vi "Main Panel.vi"(8 "error in (no error)":errorcluster) -> (0 "error out":errorcluster)   [LabVIEW 2014]
uses:
  Type'def/UPH Config.ctl
  SubVI's/VISA/Ctr/VISA Ctr.ctl
  Type'def/MainCtr.ctl
  Type'def/Main Ctr Ref.ctl
  Type'def/User Login.ctl
  <vilib>/addons/database/Connection.llb/Conn ObjectReference.ctl
  <vilib>/addons/database/NI_Database_API.lvlib
  SubVI's/Database/Ctr/Constr.ctl
  SubVI's/Database/Ctr/Conneect State.ctl
  Type'def/DB Query.ctl
  Type'def/Main FTT.ctl
  SubVI's/Simatic S7/Function/Write/Write Sigle Data/Write Sigle Bool.vi
  SubVI's/Simatic S7/Simatic S7.lvlib
  <vilib>/addons/database/_DB Variant To Data/Database Variant To Data.xnode
  Type'def/FTT Display Type.ctl
panel:
  out "ArrayStr out":string[](array[string])
  in  "Login":bool
  out "Login":T1 caption="用户登录信息"
  out "Date&Time":string
  in  "Exit":bool
  in  "Config":bool
  in  "Query DB":bool
  in  "Main Panel":bool
  in  "Table":enum32{"Main", "Database", "Config"}(tab)
  in  "Error Table":i32(listbox)
  out "Display":T2
  in  "DB Dispaly":T3 {"StartTime" format="%<%Y/%m/%d %H:%M>T"; "EndTime" format="%<%Y/%m/%d %H:%M>T"}
  in  "FTT_Submit":bool
  out "IP Address":string[](array[string])
  in  "Scaner":bool
  in  "Shield Signe":bool
  in  "UPH":bool
  in  "Modfy TV":bool
  # "Inalfa roof systems(Shanghai) CO.LT"
  # "Plan/Targe(%)"
  # "Taget/Actual"
  # "FTT/FTT(%)"
  # "Repaired/Reject"
  # "/"
  # "/"
  # "/"
  # "/"
  # "硬件配置"
  # "参数配置"
  # "其他配置"
  # "当前系统CPU地址"
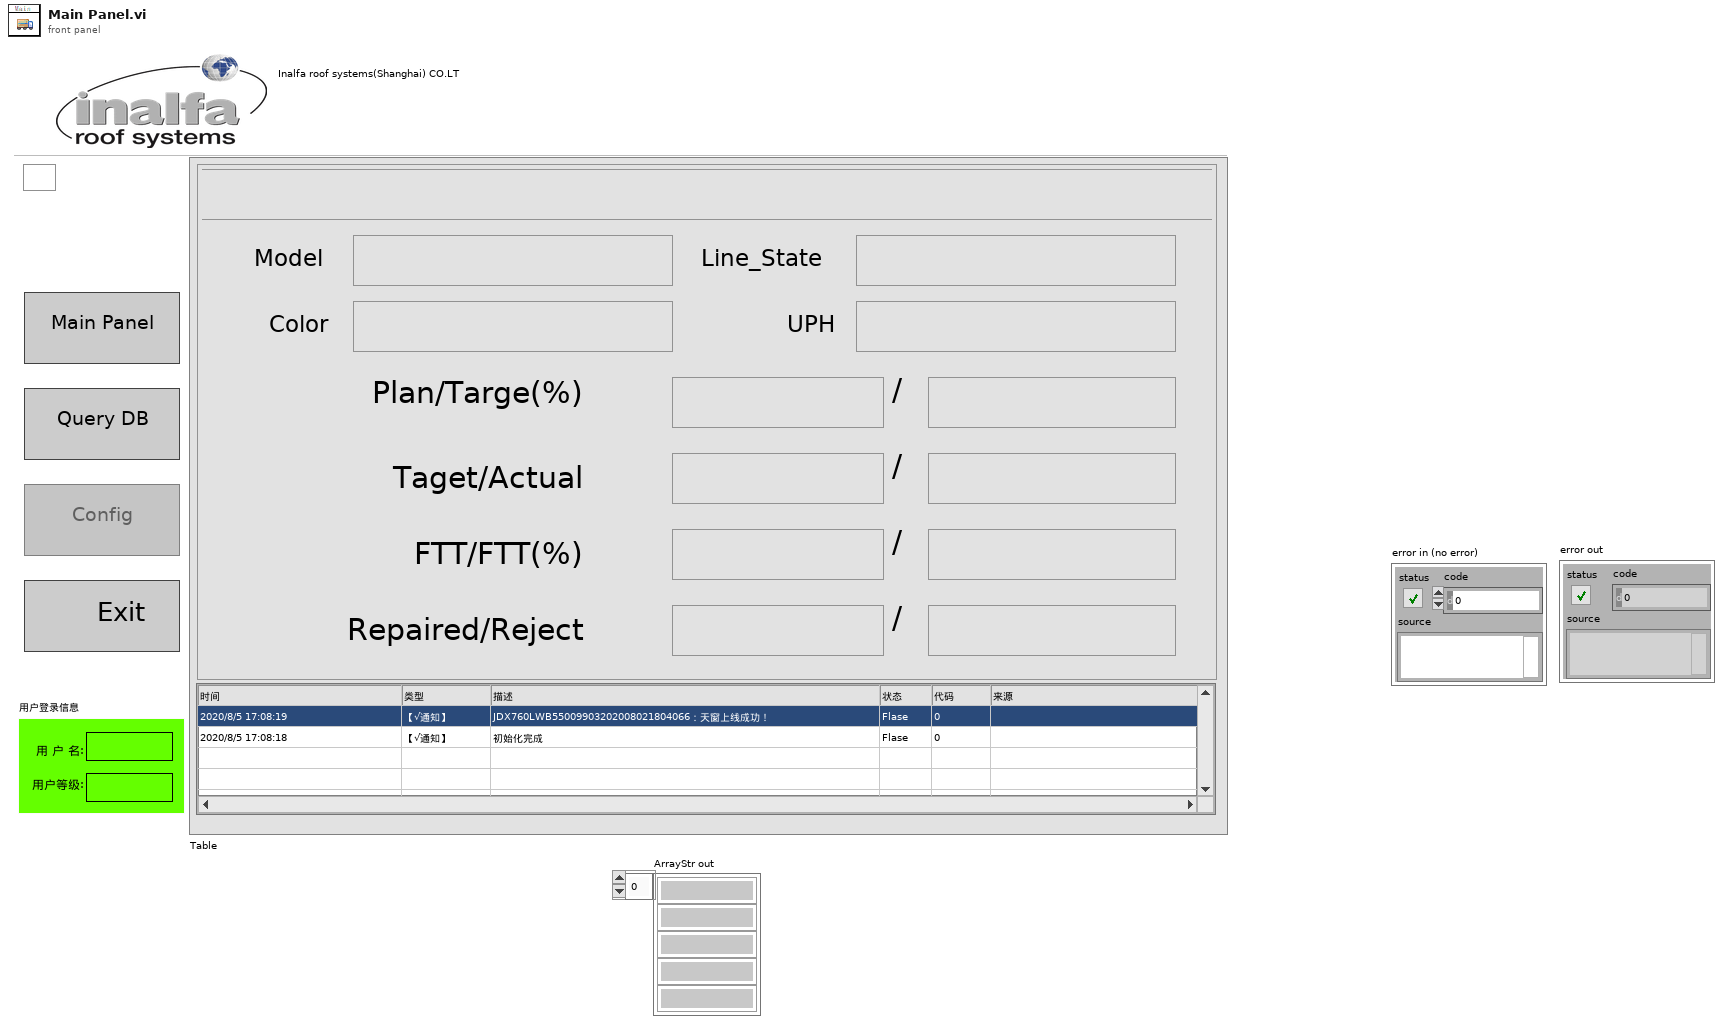
[diagram p1: front panel]
types:
  T1 = typedef "User Login.ctl" = cluster{"User":string, "Grade":string}
  T2 = typedef "Main FTT.ctl" = cluster{"Line_Name":string, "Model":string, "Line_State":string, "Color":string, "UPH":string, "Plan":string, "Target Rate":string, "Target":string, "Actual":string, "FTT":string, "FTT Rate":string, "Repaired":string, "Reject":string}
  T3 = cluster{"Export":bool, "Query":bool, "Station.No":string, "EndTime":timestamp, "StartTime":timestamp, "FTT":cluster{"FTT":string, "OutLine":string, "FTT Rata":string}, "TableName":string, "List":string[][], "Station":bool, "QTime":enum32{"Online", "Outline"}}
  T4 = typedef "MainCtr.ctl" = cluster{"Tite":string, "Base path":path, "Table":cluster{"Table":string, "alias":string}[], "Stations":cluster{"Stations":string, "alias":string}[], "Shield Array":bool[], "UPHs":T5[], "VISA":T6, "Path":cluster{"roof":path, "Config":path, "Png":path}, "Ctr":T7, "Login":T1, "information":cluster{"cause":string, "Type":enum16{"Inform", "Warning", "Alarm"}, "code":i32, "Suroce":string, "Status":bool}, "Local DB":cluster{"Connstr":string, "Database":T8}, "Remote DB":cluster{"Connstr":string, "Database":T8}, "FTT TV":string, "ExchangeTime":i32, "NVH":string, "EOL Path":path}
  T5 = typedef "UPH Config.ctl" = cluster{"Line_No":string, "Model":string, "B_UPH ":i16, "S_UPH  ":i16, "Class":enum16{"Big", "Small"}}
  T6 = typedef "VISA Ctr.ctl" = cluster{"VISA":refnum<visa-resource-name>, "baud rate":u32, "data bits":u16, "parity":enum16{"None", "Odd", "Even", "Mark", "Space"}, "stop bits":u16, "flow control":u16}
  T7 = typedef "Main Ctr Ref.ctl" = cluster{"DB Dispaly":refnum<vi>, "Error Table":refnum<vi>, "Display":refnum<vi>, "Login":refnum<vi>, "Exit":refnum<vi>, "FTT_Submit":refnum<vi>}
  T8 = typedef "Conneect State.ctl" = cluster{"Constr":T9, "conn ref":T10, "State":bool}
  T9 = typedef "Constr.ctl" = cluster{"Driver":string, "Server":string, "User":string, "Pwd":string, "Database":string}
  T10 = typedef "NI_Database_API.lvlib/Conn ObjectReference.ctl" = refnum<k1>
  T11 = enum8{"Enabled", "Disabled", "Disabled and Grayed Out"}
  T12 = typedef "DB Query.ctl" = cluster{"Export":bool, "Query":bool, "Station.No":string, "EndTime":timestamp, "StartTime":timestamp, "FTT":cluster{"FTT":string, "OutLine":string, "FTT Rata":string}, "TableName":string, "List":string[][], "Station":bool, "QTime":enum32{"Online", "Outline"}}
  T13 = typedef "FTT Display Type.ctl" = cluster{"Line.No":string, "Model":string, "Color":string, "UPH":dbl, "Plan":dbl, "Target Rate":dbl, "Target ":dbl, "Actual":dbl, "FTT":dbl, "FTT Rate":dbl, "Repaired":dbl, "Reject":dbl, "Ouline":dbl, "Line State":string}
  T14 = cluster{"Display":T13, "Class":enum16{"Big", "Small"}}
  T15 = cluster{"cause":string, "Type":enum16{"Inform", "Warning", "Alarm"}, "code":i32, "Suroce":string, "Status":bool}
  T16 = typedef "Simatic S7.lvlib/Operation Siemens Ref.ctl" = enum16{"Init", "Add Ref", "Get Ref", "Set Error", "Close Close"}
  T17 = cluster{"Base path":path, "Config path":path, "Log DB Error":path}
  T18 = cluster{"DB Dispaly":refnum<vi>, "Error Table":refnum<vi>, "Display":refnum<vi>, "Login":refnum<vi>, "Exit":refnum<vi>, "FTT_Submit":refnum<vi>}
  T19 = cluster{"Username":string, "GradeStr":string, "Grade":u32}
  T20 = typedef "Simatic S7.lvlib/Siemens Ref.ctl" = cluster{"IP Address ":string, "Conn ID":refnum<k5>, "Timeout ms":i32, "Status":bool, "Slot":u16, "Rack":u16}
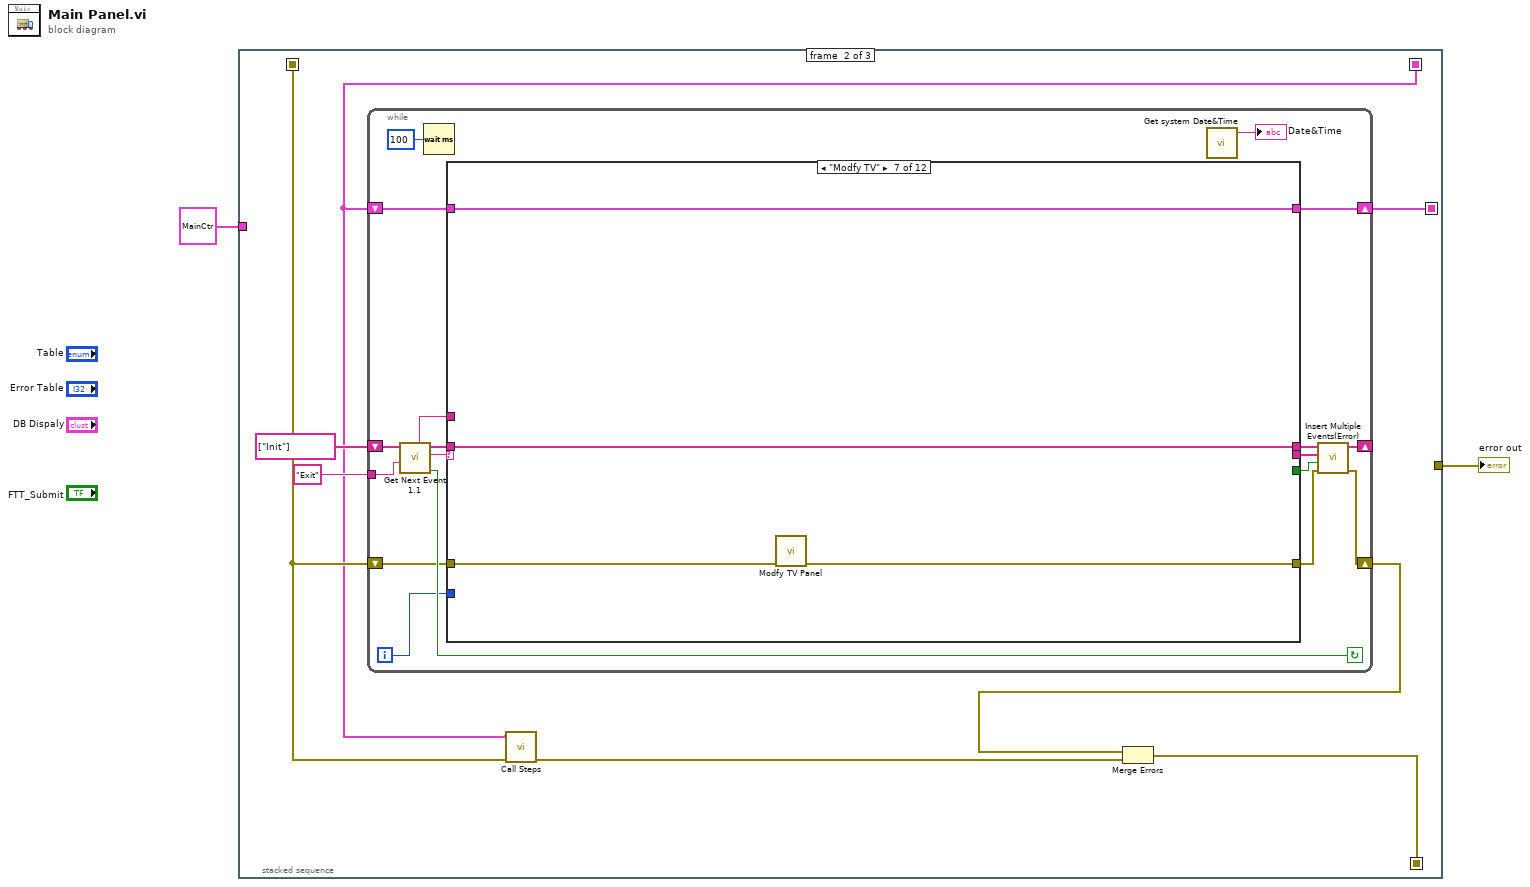
[diagram p0: block diagram]
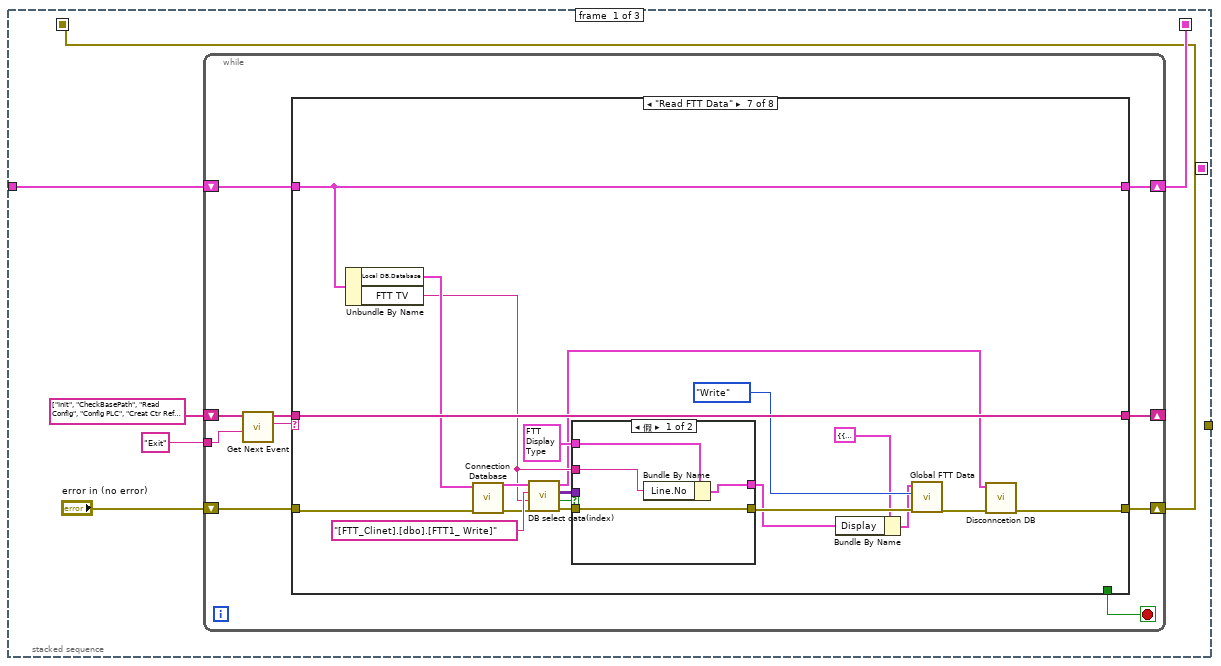
[diagram p2: hidden frame]
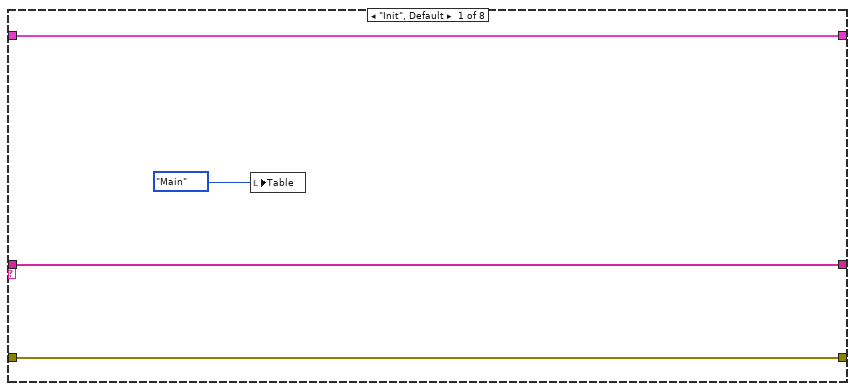
[diagram p3: hidden frame]
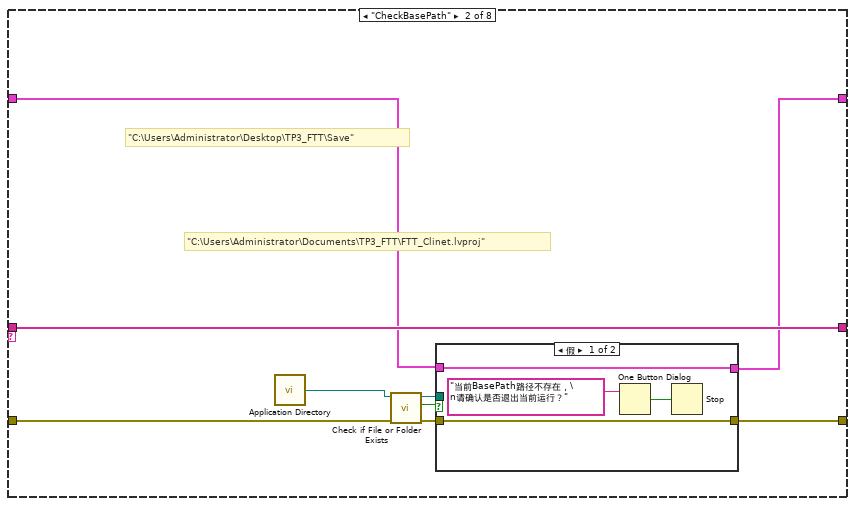
[diagram p4: hidden frame]
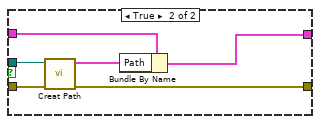
[diagram p5: hidden frame]
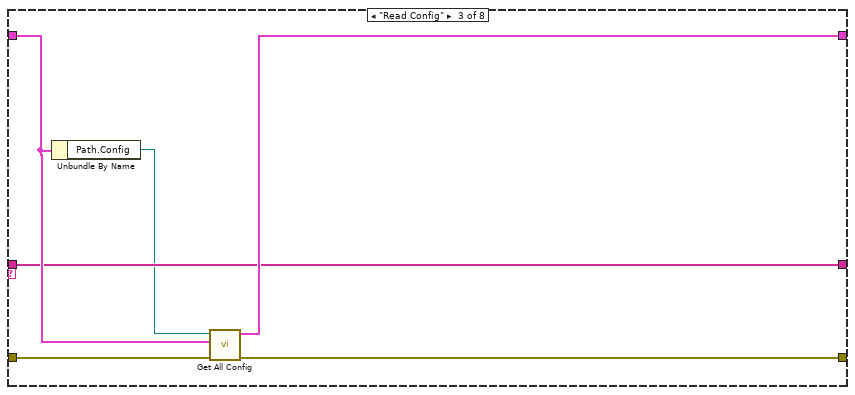
[diagram p6: hidden frame]
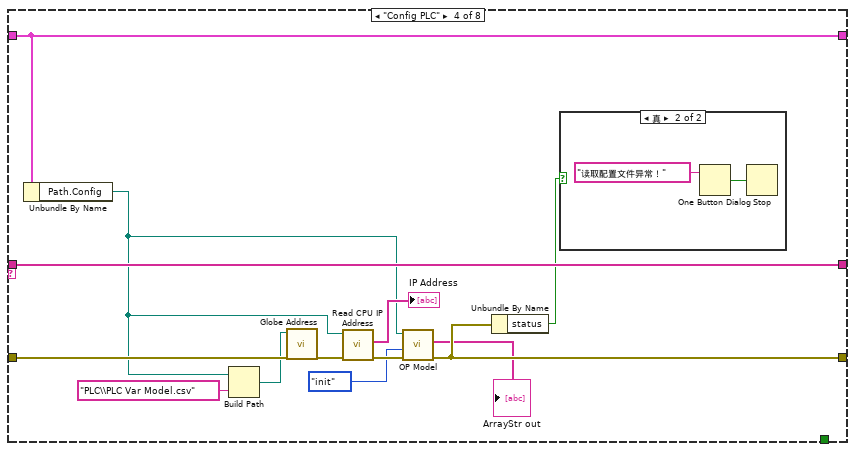
[diagram p7: hidden frame]
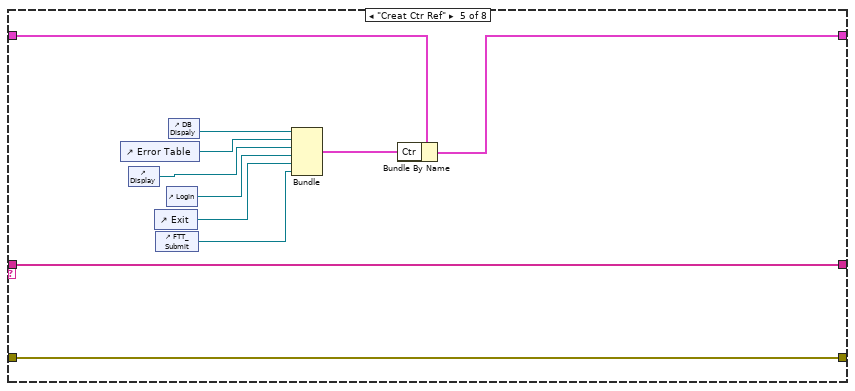
[diagram p9: hidden frame]
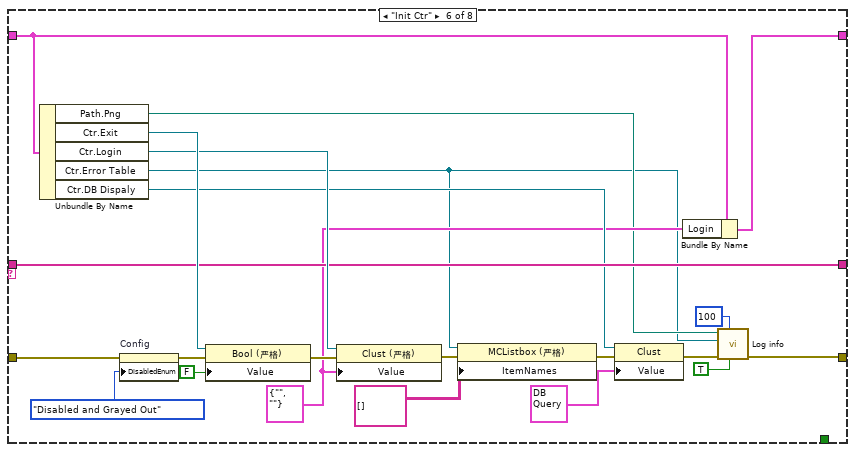
[diagram p10: hidden frame]
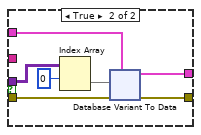
[diagram p11: hidden frame]
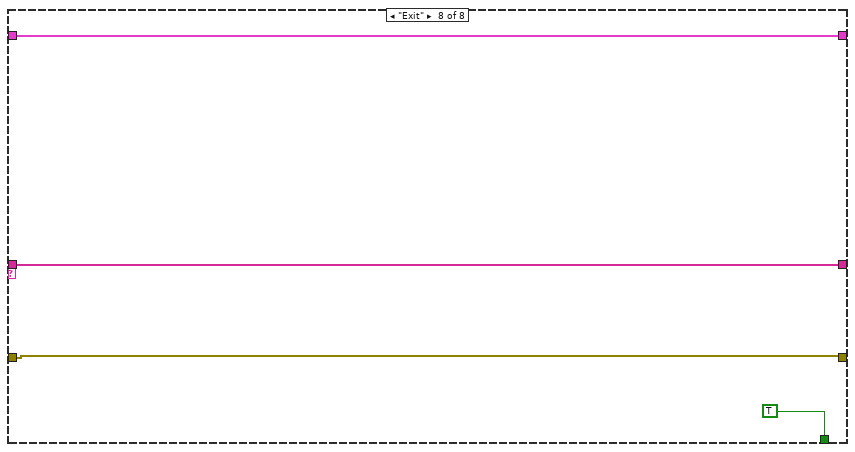
[diagram p12: hidden frame]
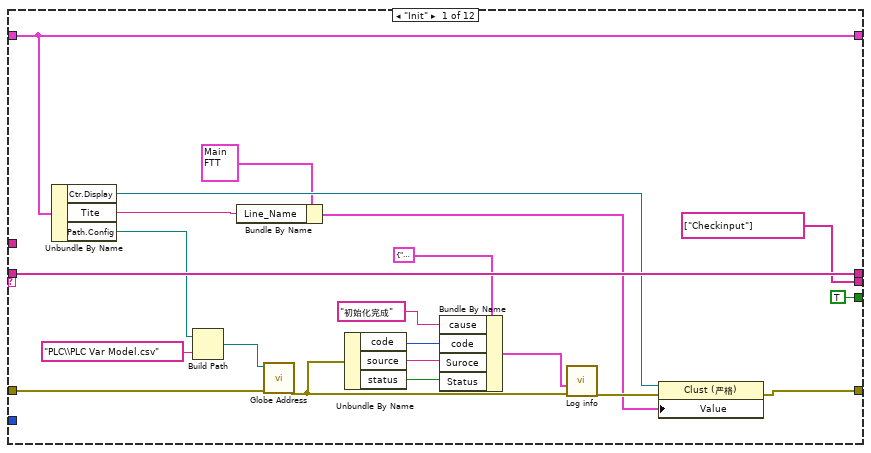
[diagram p13: hidden frame]
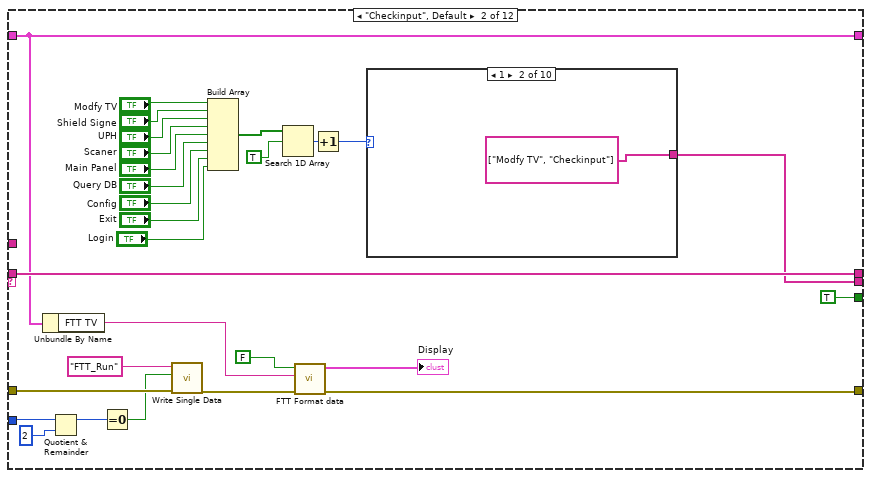
[diagram p14: hidden frame]
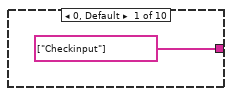
[diagram p15: hidden frame]
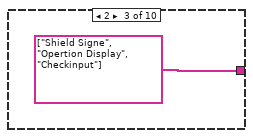
[diagram p16: hidden frame]
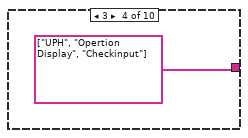
[diagram p17: hidden frame]
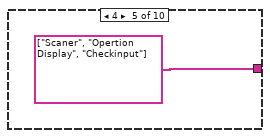
[diagram p18: hidden frame]
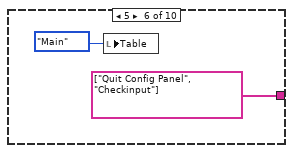
[diagram p19: hidden frame]
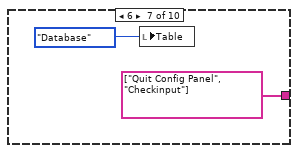
[diagram p20: hidden frame]
diagram:
  n1 = stacked-sequence {
    seq-local: [w4 _ _] -> [_ w569 _]
    seq-local: [w3 _ _] -> [_ w574 _]
    seq-local: [_ w571 _] -> [_ _ w768]
    seq-local: [_ w570 _] -> [_ _ _]
    tunnel: T4 {"Tite"="", "Base path"=path "", "Table"=[], "Stations"=[], "Shield Array"=[], "UPHs"=[], "VISA"={"VISA"="", "baud rate"=9600, "data bits"=8, "parity"=enum."None", "stop bits"=10, "flow control"=0}, "Path"={"roof"=path "", "Config"=path "", "Png"=path ""}, "Ctr"={"DB Dispaly"=refnum, "Error Table"=refnum, "Display"=refnum, "Login"=refnum, "Exit"=refnum, "FTT_Submit"=refnum}, "Login"={"User"="", "Grade"=""}, "information"={"cause"="", "Type"=enum."Inform", "code"=0, "Suroce"="", "Status"=FALSE}, "Local DB"={"Connstr"="", "Database"={"Constr"={"Driver"="", "Server"="", "User"="", "Pwd"="", "Database"=""}, "conn ref"=refnum, "State"=FALSE}}, "Remote DB"={"Connstr"="", "Database"={"Constr"={"Driver"="", "Server"="", "User"="", "Pwd"="", "Database"=""}, "conn ref"=refnum, "State"=FALSE}}, "FTT TV"="", "ExchangeTime"=0, "NVH"="", "EOL Path"=path ""} ("Cluster") -> [w6 _ _]
    tunnel: [_ _ w762] -> w1
    frame #0 {
      n2 = while {
        shift-right: [w13] -> _
        shift-left: string[] ["Init", "CheckBasePath", "Read Config", "Config PLC", "Creat Ctr Ref", "Read FTT Data", "Init Ctr", "Exit"] -> [w18]
        tunnel: "Exit" ("Exit Event") -> [w15]
        shift-right: [w10] -> w4
        shift-left: w6 -> [w14]
        shift-right: [w11] -> w3
        shift-left: "error in (no error)" -> [w12]
        stop <- w9 stop-if-true
        n3 = call "Get Next Event.vi"("Exit Event"=w15, "event queue in"=w18) -> ("next event"=w17:string, "event queue out"=w16:string[])  [unwired: 3 in, 1 out]
        n4 = case shown="\"Read FTT Data\"" w17 {
          tunnel: w16 -> [w21 w31 w44 w55 w73 w89 w115 w567]
          tunnel: w14 -> [w22 w26 w46 w59 w67 w85 w99 w566]
          tunnel: [w21 w31 w44 w55 w73 w89 w115 w567] -> w13
          tunnel: w12 -> [w20 w30 w47 w58 w72 w76 w106 w565]
          tunnel: [w20 w25 w42 w51 w72 w81 w100 w565] -> w11
          tunnel: [w22 w24 w45 w59 w66 w84 w99 w566] -> w10
          tunnel: [_ _ _ _ _ _ _ TRUE] -> w9
          frame "Init", Default {
            n5 = local write "Table"(enum32{"Main", "Database", "Config"}."Main" ("Table")) -> ()
          }
          frame "CheckBasePath" {
            # "\"C:\\Users\\Administrator\\Documents\\TP3_FTT\\FTT_Clinet.lvproj\""
            # "\"C:\\Users\\Administrator\\Desktop\\TP3_FTT\\Save\""
            n6 = call <vilib>:"Application Directory.vi"() -> ("Application Directory"=w23:path)
            n7 = call <vilib>:"Check if File or Folder Exists.vi"("error in (no error)"=w30, "path"=w23) -> ("error out"=w28:errorcluster, "file or folder exists?"=w29:bool, "dup path"=w27:path)  [unwired: 7 in]
            n8 = case shown="假" w29 {
              tunnel: w28 -> [w35 w41]
              tunnel: w27 -> [_ w40]
              tunnel: w26 -> [w34 w39]
              tunnel: [w35 w37] -> w25
              tunnel: [w34 w36] -> w24
              frame False {
                n9 = One Button Dialog(message="当前BasePath路径不存在，\n请确认是否退出当前运行？") -> (true=w33:bool)  [unwired: 1 in]
                n10 = Stop(stop? (T)=w33) -> ()
              }
              frame True {
                n11 = call "Creat Path.vi"("error in (no error)"=w41, "base path"=w40) -> ("error out"=w37:errorcluster, "output cluster"=w38:T17)  [unwired: 8 in]
                n12 = Bundle By Name(cluster=w39, "Path"=w38) -> (w36:T4)
              }
            }
          }
          frame "Read Config" {
            n13 = Unbundle By Name(w46) -> ("Path.Config"=w43:path)
            n14 = call "Get All Config.vi"("error in (no error)"=w47, "Main Ctr in"=w46, "Base Path"=w43) -> ("error out"=w42:errorcluster, "Cluster"=w45:T4)  [unwired: 7 in]
          }
          frame "Config PLC" {
            n15 = Unbundle By Name(w59) -> ("Path.Config"=w49:path)
            n16 = Build Path(base path=w49, name or relative path="PLC\\PLC Var Model.csv") -> (appended path=w57:path)
            n17 = call "Globe Address.vi"("error in (no error)"=w58, "file path (dialog if empty)"=w57) -> ("error out"=w56:errorcluster)  [unwired: 6 in, 3 out]
            n18 = call "Read CPU IP Address.vi"("error in (no error)"=w56, "base path"=w49) -> ("error out"=w52:errorcluster, "IP Address"=→"IP Address":string[])  [unwired: 7 in, 1 out]
            n19 = call "OP Model.vi"("error in (no error)"=w52, "Enum"=enum16{"init", "Read", "Write"}."init", "Path"=w49) -> ("error out"=w51:errorcluster, "ArrayStr out"=→"ArrayStr out":string[])  [unwired: 6 in, 1 out]
            n20 = Unbundle By Name(w51) -> ("status"=w53:bool)
            n21 = case shown="真" w53 {
              frame False {
              }
              frame True {
                n22 = One Button Dialog(message="读取配置文件异常！") -> (true=w61:bool)  [unwired: 1 in]
                n23 = Stop(stop? (T)=w61) -> ()
              }
            }
          }
          frame "Creat Ctr Ref" {
            n24 = control-ref of="Error Table"() -> (w69:refnum<vi>)
            n25 = control-ref of="Display"() -> (w65:refnum<vi>)
            n26 = control-ref of="Exit"() -> (w71:refnum<vi>)
            n27 = control-ref of="FTT_Submit"() -> (w64:refnum<vi>)
            n28 = control-ref of="Login"() -> (w70:refnum<vi>)
            n29 = control-ref of="DB Dispaly"() -> (w68:refnum<vi>)
            n30 = Bundle("DB Dispaly"=w68, "Error Table"=w69, "Display"=w65, "Login"=w70, "Exit"=w71, "FTT_Submit"=w64) -> (w63:T18)  [unwired: 1 in]
            n31 = Bundle By Name(cluster=w67, "Ctr"=w63) -> (w66:T4)
          }
          frame "Init Ctr" {
            w83 = T1 {"User"="", "Grade"=""} ("Value")
            n32 = Unbundle By Name(w85) -> ("Path.Png"=w80:path, "Ctr.Exit"=w95:refnum<vi>, "Ctr.Login"=w92:refnum<vi>, "Ctr.Error Table"=w79:refnum<vi>, "Ctr.DB Dispaly"=w87:refnum<vi>)
            n33 = property on="Config" class="Bool"(error in=w76, "DisabledEnum"=T11."Disabled and Grayed Out" ("Disabled")) -> (error out=w75:errorcluster)  [unwired: 1 in, 1 out]
            n34 = property class="Bool (严格)"(reference=w95, error in=w75, "Value"=FALSE) -> (error out=w93:errorcluster)  [unwired: 1 out]
            n35 = property class="Clust (严格)"(reference=w92, error in=w93, "Value"=w83) -> (error out=w91:errorcluster)  [unwired: 1 out]
            n36 = property class="MCListbox (严格)"(reference=w79, error in=w91, "ItemNames"=string[][] [] ("Value")) -> (error out=w88:errorcluster)  [unwired: 1 out]
            n37 = property class="Clust"(reference=w87, error in=w88, "Value"=T12 {"Export"=FALSE, "Query"=FALSE, "Station.No"="", "EndTime"=timestamp(0 s since 1904-01-01), "StartTime"=timestamp(0 s since 1904-01-01), "FTT"={"FTT"="", "OutLine"="", "FTT Rata"=""}, "TableName"="", "List"=[], "Station"=FALSE, "QTime"=enum."Online"} ("DB Dispaly")) -> (error out=w82:errorcluster)  [unwired: 1 out]
            n38 = Bundle By Name(cluster=w85, "Login"=w83) -> (w84:T4)
            n39 = call "Log info.vi"("Ref ?"=TRUE, "Rows"=100, "error in (no error)"=w82, "MCListbox引用句柄"=w79, "Base"=w80) -> ("error out"=w81:errorcluster)  [unwired: 5 in, 1 out]
          }
          frame "Read FTT Data" {
            n40 = Unbundle By Name(w99) -> ("Local DB.Database"=w107:T8, "FTT TV"=w105:string)
            n41 = call "Connection Database.vi"("error in (no error)"=w106, "Connncet State"=w107) -> ("error out"=w109:errorcluster, "Connncet State out"=w108:T8)  [unwired: 8 in]
            n42 = call "DB select data(index).vi"("error in (no error)"=w109, "Code"=w105, "Tabe"="[FTT_Clinet].[dbo].[FTT1_ Write]", "Connncet State"=w108) -> ("error out"=w112:errorcluster, "state"=w113:bool, "data"=w111:variant[][], "Connncet State out"=w101:T8)  [unwired: 4 in]
            n43 = case shown="假" w113 {
              tunnel: w112 -> [w119 w124]
              tunnel: w111 -> [_ w126]
              tunnel: T13 {"Line.No"="", "Model"="", "Color"="", "UPH"=0.0, "Plan"=0.0, "Target Rate"=0.0, "Target "=0.0, "Actual"=0.0, "FTT"=0.0, "FTT Rate"=0.0, "Repaired"=0.0, "Reject"=0.0, "Ouline"=0.0, "Line State"=""} ("Display") -> [w118 w122]
              tunnel: [w119 w121] -> w104
              tunnel: [w116 w120] -> w97
              tunnel: w105 -> [w117 _]
              frame False {
                n44 = Bundle By Name(cluster=w118, "Line.No"=w117) -> (w116:T13)
              }
              frame True {
                n45 = Index Array(array=w126, index (row)=0) -> (element=w123:variant[])  [unwired: 1 in]
                n46 = xnode "Database Variant To Data"("database variant"=w123, "error in (no error)"=w124, "type"=w122) -> ("data"=w120:T13, "error out"=w121:errorcluster)
              }
            }
            n47 = Bundle By Name(cluster=T14 {"Display"={"Line.No"="", "Model"="", "Color"="", "UPH"=0.0, "Plan"=0.0, "Target Rate"=0.0, "Target "=0.0, "Actual"=0.0, "FTT"=0.0, "FTT Rate"=0.0, "Repaired"=0.0, "Reject"=0.0, "Ouline"=0.0, "Line State"=""}, "Class"=enum."Big"} ("Display"), "Display"=w97) -> (w96:T14)
            n48 = call "Global FTT Data.vi"("error in (no error)"=w104, "Mode"=enum16{"Read", "Write"}."Write", "Display"=w96) -> ("error out"=w102:errorcluster)  [unwired: 7 in, 1 out]
            n49 = call "Disconncetion DB.vi"("error in (no error)"=w102, "Connncet State"=w101) -> ("error out"=w100:errorcluster)  [unwired: 8 in, 1 out]
          }
          frame "Exit" {
          }
        }
      }
    }
    frame #1 {
      n50 = while {
        shift-right: [w587] -> _
        shift-left: string[] ["Init"] ("event queue out") -> [w591]
        tunnel: "Exit" ("Exit Event") -> [w588]
        shift-right: [w579] -> w572
        shift-left: w574 -> [w578]
        shift-right: [w582] -> w570
        shift-left: w569 -> [w583]
        i -> [w581]
        stop <- w589 continue-if-true
        n51 = call "Get Next Event 1.1.vi"("Exit Event"=w588, "event queue in"=w591) -> ("Condition (Exit:F)"=w589:bool, "next event"=w592:string, "event queue out"=w590:string[], "Previous Event"=w577:string)  [unwired: 6 in]
        n52 = Wait (ms)(milliseconds to wait=u32 100) -> ()  [unwired: 1 out]
        n53 = case shown="\"Modfy TV\"" w592 {
          tunnel: w590 -> [w615 w643 w668 w686 w701 w711 w722 w727 w737 w746 _ _]
          tunnel: [w615 w643 w668 w686 w701 w711 w722 w727 w737 w746 _ w760] -> w586
          tunnel: [TRUE TRUE _ _ _ _ _ _ _ _ FALSE FALSE] -> w585
          tunnel: [string[] ["Checkinput"] ("event queue out") w629 _ _ _ _ _ _ _ _ string[] ["Checkinput"] ("event queue out") _] -> w584
          tunnel: w578 -> [w612 w628 w670 w685 w702 w713 w724 w726 w735 w741 w750 w757]
          tunnel: [w596 w617 w662 w678 w696 w707 w723 w726 w730 w745 w749 w753] -> w580
          tunnel: w583 -> [w595 w620 w656 w680 w692 w710 w725 w728 w736 w744 w751 w756]
          tunnel: [w595 w620 w656 w679 w691 w709 w725 w728 w736 w744 w751 w756] -> w582
          tunnel: w581 -> [_ w627 _ _ _ _ _ _ _ _ _ _]
          tunnel: w577 -> [_ _ _ _ _ _ _ _ _ _ _ _]
          frame "Init" {
            n54 = Unbundle By Name(w595) -> ("Ctr.Display"=w600:refnum<vi>, "Tite"=w598:string, "Path.Config"=w611:path)
            n55 = Build Path(base path=w611, name or relative path="PLC\\PLC Var Model.csv") -> (appended path=w610:path)
            n56 = Bundle By Name(cluster=T2 {"Line_Name"="", "Model"="", "Line_State"="", "Color"="", "UPH"="", "Plan"="", "Target Rate"="", "Target"="", "Actual"="", "FTT"="", "FTT Rate"="", "Repaired"="", "Reject"=""} ("Value"), "Line_Name"=w598) -> (w597:T2)
            n57 = call "Globe Address.vi"("error in (no error)"=w612, "file path (dialog if empty)"=w610) -> ("error out"=w606:errorcluster)  [unwired: 6 in, 3 out]
            n58 = Unbundle By Name(w606) -> ("code"=w603:i32, "source"=w604:string, "status"=w605:bool)
            n59 = Bundle By Name(cluster=T15 {"cause"="我问问", "Type"=enum."Inform", "code"=0, "Suroce"="", "Status"=FALSE} ("information"), "cause"="初始化完成" ("Suroce"), "code"=w603, "Suroce"=w604, "Status"=w605) -> (w607:T15)
            n60 = call "Log info.vi"("error in (no error)"=w606, "information"=w607) -> ("error out"=w601:errorcluster)  [unwired: 8 in, 1 out]
            n61 = property class="Clust (严格)"(reference=w600, error in=w601, "Value"=w597) -> (error out=w596:errorcluster)  [unwired: 1 out]
          }
          frame "Checkinput", Default {
            n62 = Unbundle By Name(w620) -> ("FTT TV"=w619:string)
            n63 = Quotient & Remainder(x=w627, y=2) -> (x-y*floor(x/y)=w625:i32)  [unwired: 1 out]
            n64 = Equal To 0?(x=w625) -> (x = 0?=w624:bool)
            n65 = call-poly "Write Single Data.vi"("error in (no error)"=w628, "Data"=w624, "Tags"="FTT_Run") -> ("error out"=w622:errorcluster)  [unwired: 6 in, 2 out]
            n66 = Build Array("Modfy TV", "Shield Signe", "UPH", "Scaner", "Main Panel", "Query DB", "Config", "Exit", "Login") -> (w633:bool[])
            n67 = Search 1D Array(1D array=w633, element=TRUE) -> (index of element=w631:i32)  [unwired: 1 in]
            n68 = call "FTT Format data.vi"("error in (no error)"=w622, "FTT_TV"=w619, "W/R"=FALSE) -> ("error out"=w617:errorcluster, "Display"=→"Display":T2)  [unwired: 6 in, 1 out]
            n69 = Increment(x=w631) -> (x+1=w630:i32)
            n70 = case shown="1" w630 {
              tunnel: [string[] ["Checkinput"] ("event queue out") string[] ["Modfy TV", "Checkinput"] string[] ["Shield Signe", "Opertion Display", "Checkinput"] string[] ["UPH", "Opertion Display", "Checkinput"] string[] ["Scaner", "Opertion Display", "Checkinput"] string[] ["Quit Config Panel", "Checkinput"] string[] ["Quit Config Panel", "Checkinput"] string[] ["Config Panel", "Checkinput"] string[] ["Quit"] ("event queue out") string[] ["User Log", "Checkinput"]] -> w629
              frame 0, Default {
              }
              frame 1 {
              }
              frame 2 {
              }
              frame 3 {
              }
              frame 4 {
              }
              frame 5 {
                n71 = local write "Table"(enum32{"Main", "Database", "Config"}."Main" ("Table")) -> ()
              }
              frame 6 {
                n72 = local write "Table"(enum32{"Main", "Database", "Config"}."Database" ("Table")) -> ()
              }
              frame 7 {
              }
              frame 8 {
              }
              frame 9 {
              }
            }
          }
          frame "User Log" {
            n73 = Unbundle By Name(w656) -> ("Path.Config"=w669:path)  [unwired: 1 out]
            n74 = call "User and Password.vi"("error in (no error)"=w670, "Path"=w669) -> ("error out"=w663:errorcluster, "output cluster"=w667:T19)  [unwired: 8 in]
            n75 = Unbundle By Name(w667) -> ("Username"=w666:string, "GradeStr"=w665:string, "Grade"=w661:u32)
            n76 = Greater Than 0?(x=w661) -> (x > 0?=w659:bool)
            n77 = Bundle("Username"=w666, "GradeStr"=w665) -> (→"Login":cluster{"Username":string, "GradeStr":string})  [unwired: 1 in]
            n78 = Select(t=T11."Enabled" ("Disabled"), s=w659, f=T11."Disabled and Grayed Out" ("Disabled")) -> (s? t:f=w660:T11)
            n79 = property on="Config" class="Bool"(error in=w663, "DisabledEnum"=w660) -> (error out=w662:errorcluster)  [unwired: 1 in, 1 out]
          }
          frame "UPH" {
            n80 = Unbundle By Name(w680) -> ("UPHs"=w676:T5[], "Path.Config"=w681:path)
            n81 = call "OP UPH Config.vi"("error in (no error)"=w685, "Enum"=enum16{"init", "Read", "Write"}."Read") -> ("error out"=w683:errorcluster, "UPH out"=w682:T5[])  [unwired: 7 in, 1 out]
            n82 = call "UPH Panel.vi"("error in (no error)"=w683, "Base path"=w681, "UPH in"=w682) -> ("error out"=w678:errorcluster, "UPH out"=w677:T5[])  [unwired: 7 in]
            n83 = Unbundle By Name(w678) -> ("status"=w674:bool)
            n84 = Select(t=w676, s=w674, f=w677) -> (s? t:f=w675:T5[])
            n85 = Select(t="UPH修改保存异常！", s=w674, f="UPH修改保存成功！") -> (s? t:f=w673:string)
            n86 = Bundle By Name(cluster=w680, "UPHs"=w675, "information.cause"=w673) -> (w679:T4)
          }
          frame "Scaner" {
            n87 = Unbundle By Name(w692) -> ("VISA"=w694:T6, "Path.Config"=w697:path)
            n88 = call "OP Scaner Config.vi"("error in (no error)"=w702, "Enum"=enum16{"init", "Read", "Write"}."Read") -> ("error out"=w699:errorcluster, "VISA"=w698:T6)  [unwired: 7 in, 1 out]
            n89 = call "Scaner Panel.vi"("error in (no error)"=w699, "VISA in"=w698, "Base path"=w697) -> ("error out"=w696:errorcluster, "VISA out"=w695:T6)  [unwired: 7 in]
            n90 = Unbundle By Name(w696) -> ("status"=w690:bool)
            n91 = Select(t=w694, s=w690, f=w695) -> (s? t:f=w693:T6)
            n92 = Select(t="Scaner修改保存异常！", s=w690, f="Scaner修改保存成功！") -> (s? t:f=w689:string)
            n93 = Bundle By Name(cluster=w692, "VISA"=w693, "information.cause"=w689) -> (w691:T4)
          }
          frame "Shield Signe" {
            w706 = enum16{"init", "Read", "Write"}."Read" ("Enum")
            n94 = Unbundle By Name(w710) -> ("Shield Array"=w719:bool[], "Path.Config"=w720:path, "Stations"=w704:cluster{"Stations":string, "alias":string}[])
            n95 = call "OP Shield Config.vi"("error in (no error)"=w713, "Enum"=w706) -> ("error out"=w721:errorcluster, "Shield out"=w712:u32)  [unwired: 6 in, 2 out]
            n96 = call "Ger All Station Alias Name.vi"("Stations"=w704) -> ("Array"=w703:string[])  [unwired: 10 in]
            n97 = call "Station Shiled Panel.vi"("error in (no error)"=w721, "Station Name"=w703, "Base Path"=w720, "Shield"=w712) -> ("error out"=w708:errorcluster)  [unwired: 6 in, 1 out]
            n98 = call "OP Shield Config.vi"("error in (no error)"=w708, "Enum"=w706) -> ("error out"=w707:errorcluster, "subarray"=w705:bool[])  [unwired: 6 in, 2 out]
            n99 = Unbundle By Name(w707) -> ("status"=w717:bool)
            n100 = Select(t=w719, s=w717, f=w705) -> (s? t:f=w718:bool[])
            n101 = Select(t="Shield Signal修改保存异常！", s=w717, f="Shield Signal修改保存成功！") -> (s? t:f=w716:string)
            n102 = Bundle By Name(cluster=w710, "Shield Array"=w718, "information.cause"=w716) -> (w709:T4)
          }
          frame "Modfy TV" {
            n103 = call "Modfy TV Panel.vi"("error in (no error)"=w724) -> ("error out"=w723:errorcluster)  [unwired: 10 in]
          }
          frame "Config Panel" {
            n104 = local write "Table"(enum32{"Main", "Database", "Config"}."Config" ("Table")) -> ()
          }
          frame "Quit Config Panel" {
            n105 = Unbundle By Name(w736) -> ("Stations"=w734:cluster{"Stations":string, "alias":string}[], "Table"=w732:cluster{"Table":string, "alias":string}[], "Ctr.DB Dispaly"=w733:refnum<vi>, "FTT TV"=w731:string)
            n106 = call "DB Panel init.vi"("Stations"=w734, "error in (no error)"=w735, "Line_Name"=w731, "Table"=w732, "Ctr.DB Dispaly"=w733) -> ("error out"=w730:errorcluster)  [unwired: 6 in]
          }
          frame "Opertion Display" {
            n107 = Unbundle By Name(w741) -> ("status"=w740:bool, "code"=w739:i32, "source"=w738:string)
            n108 = Unbundle By Name(w744) -> ("information"=w743:T15)
            n109 = Bundle By Name(cluster=w743, "Status"=w740, "code"=w739, "Suroce"=w738) -> (w742:T15)
            n110 = call "Log info.vi"("error in (no error)"=w741, "information"=w742) -> ("error out"=w745:errorcluster)  [unwired: 8 in, 1 out]
          }
          frame "Error Log" {
            n111 = call <vilib>:"Clear Errors.vi"("error in (no error)"=w750) -> ("error out"=w749:errorcluster)  [unwired: 5 in, 1 out]
          }
          frame "Quit" {
            n112 = call "Display Message to User"("error in (no error)"=w757) -> ("error out"=w755:errorcluster, "OK"=w752:bool)  [unwired: 9 in]
            n113 = Unbundle By Name(w756) -> ("Ctr.Exit"=w754:refnum<vi>)
            n114 = property class="Bool (严格)"(reference=w754, error in=w755, "Value"=w752) -> (error out=w753:errorcluster)  [unwired: 1 out]
            n115 = Select(t=string[] ["Exit"] ("event queue out"), s=w752, f=string[] ["Checkinput"] ("event queue out")) -> (s? t:f=w760:string[])
          }
        }
        n116 = call "Get system Date&Time.vi"() -> ("date/time string"=→"Date&Time":string)  [unwired: 5 in]
        n117 = call "Insert Multiple Events(Error).vi"("error in (no error)"=w580, "Insert all? (T)"=w585, "Events to Insert"=w584, "Event queue in"=w586) -> ("error out"=w579:errorcluster, "Event queue out"=w587:string[])  [unwired: 6 in]
      }
      n118 = call "Call Steps.vi"("error in (no error)"=w574, "Cluster"=w569) -> ("error out"=w573:errorcluster)  [unwired: 9 in]
      n119 = Merge Errors(w572, w573) -> (w571:errorcluster)
    }
    frame #2 {
      n120 = call "Log info.vi"("error in (no error)"=w768, "information"=T15 {"cause"="退出当前程序！", "Type"=enum."Inform", "code"=0, "Suroce"="", "Status"=FALSE}) -> ("error out"=w766:errorcluster)  [unwired: 8 in, 1 out]
      n121 = call "Global PLC Ref.vi"("error in (no error)"=w766, "Operation Siemens Ref"=Operation_Siemens_Ref."Get Ref") -> ("error out"=w764:errorcluster, "PLC Ref"=w763:T20[])  [unwired: 5 in, 3 out]
      n122 = for {
        tunnel: w764 -> [w771]
        tunnel: w763 -> [w770] mode=indexing
        tunnel: [w769] -> w762
        n123 = call "Disconnection Siemens CPU.vi"("error in (no error)"=w771, "Siemens Ctr in"=w770) -> ("error out"=w769:errorcluster)  [unwired: 8 in, 1 out]
      }
    }
  }
  "error out" <- w1
